vi "Get Player Names and Chip Counts.vi"(11 "Hand History String in":string) -> (1 "End of players = -1":i32, 2 "Chip Count":dbl, 3 "Hand History String out":string, 4 "Player":string)   [LabVIEW 2021]
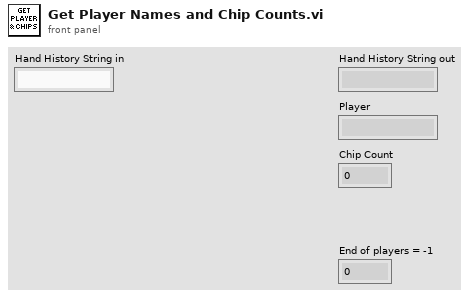
[diagram p1: front panel]
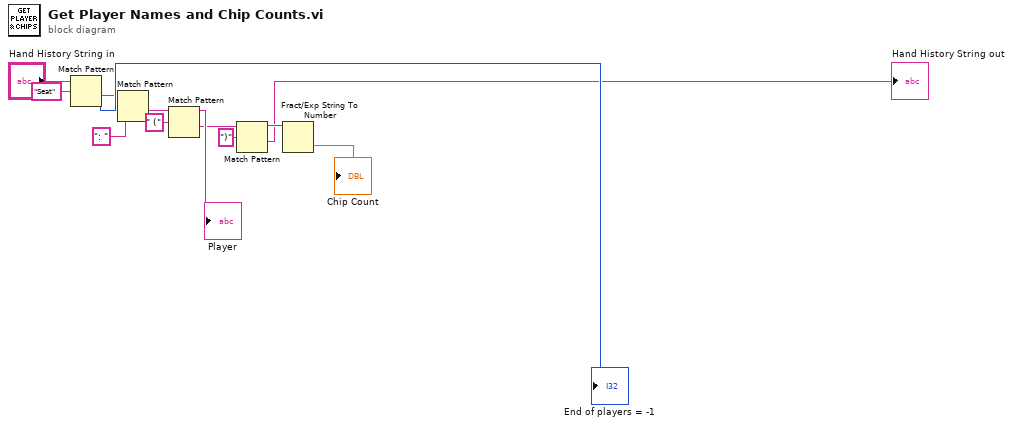
[diagram p0: block diagram]
diagram:
  n1 = Match Pattern(string="Hand History String in", regular expression="Seat") -> (after substring=w2:string, offset past match=→"End of players = -1":i32)  [unwired: 1 in, 2 out]
  n2 = Match Pattern(string=w2, regular expression=": ") -> (after substring=w4:string)  [unwired: 1 in, 3 out]
  n3 = Match Pattern(string=w4, regular expression=" (") -> (before substring=→"Player":string, after substring=w6:string)  [unwired: 1 in, 2 out]
  n4 = Match Pattern(string=w6, regular expression=")") -> (before substring=w9:string, after substring=→"Hand History String out":string)  [unwired: 1 in, 2 out]
  n5 = Fract/Exp String To Number(string=w9) -> (number=→"Chip Count":dbl)  [unwired: 3 in, 1 out]
